vi "SaveReadoutToHDF5.vi"(7 "det_hardware":enum16{"CAMERA", "PMT"}(ring), 8 "error in":errorcluster, 9 "string seq in":string, 10 "readout":T1, 11 "File Paths":T2={"Local Save Path"=path "\\\\smbhome.uscs.susx.ac.uk\\cv222/Desktop/data", "Newton Save Path"=path "Z:/#Projects/Entanglement/data", "File Name"="test", "LocalSave"=TRUE}) -> (0 "error out":errorcluster, 3 "New data?":bool=TRUE)   [LabVIEW 2019]
uses:
  controls/FilePaths.ctl
  controls/GlobalExp.vi
  Global.lvlib
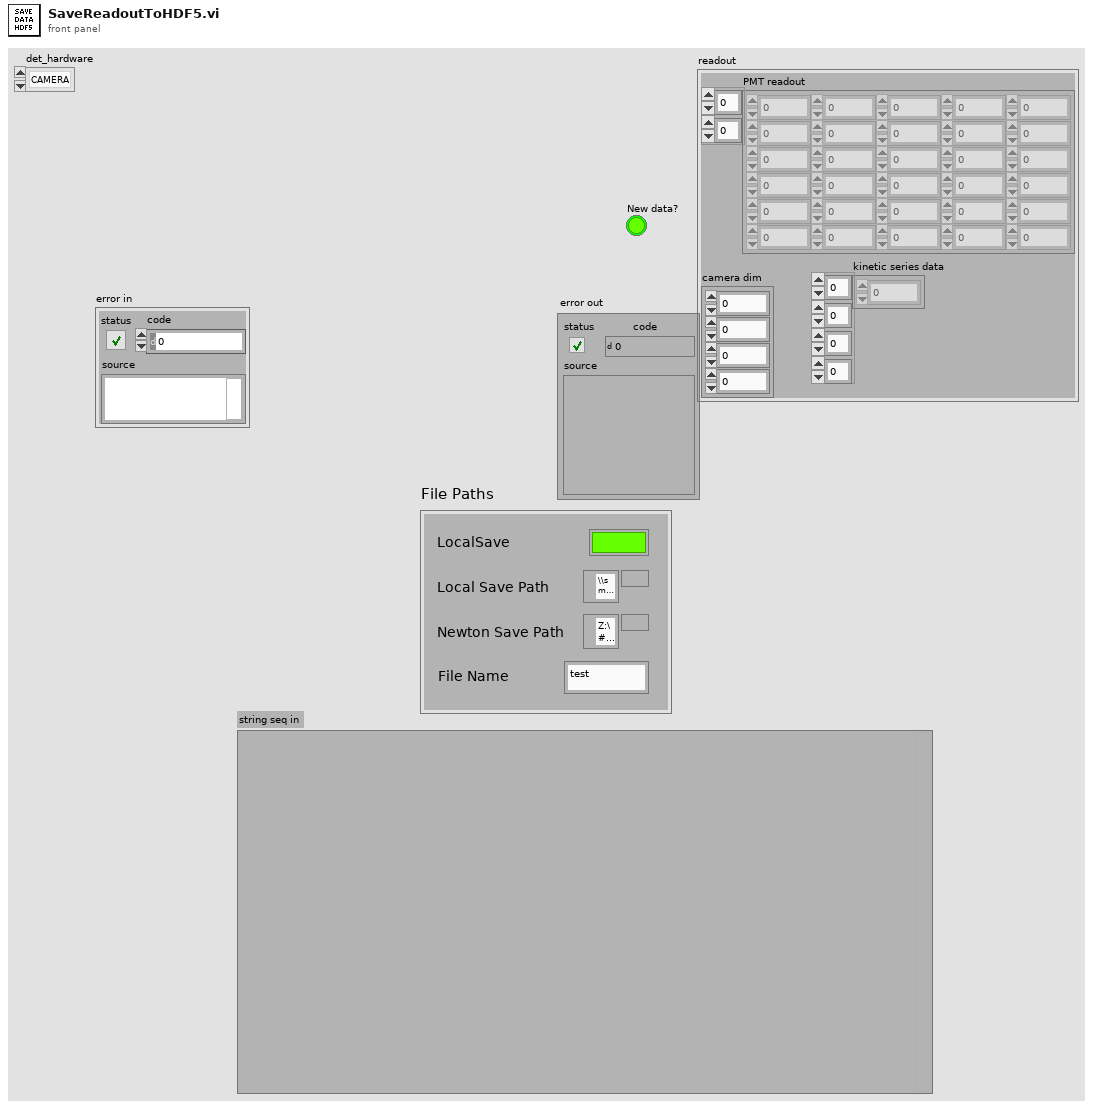
[diagram p1: front panel]
types:
  T1 = cluster{"PMT readout":u32[][], "kinetic series data":i32[][][][], "camera dim":cluster{i32, i32, i32, i32}}
  T2 = typedef "FilePaths.ctl" = cluster{"Local Save Path":path, "Newton Save Path":path, "File Name":string, "LocalSave":bool}
  T3 = cluster{"command":string, "steps":dbl, "runs":dbl, "det_hardware":string, "mathematica":string, "cam_dim":cluster{i32, i32, i32, i32}}
  T4 = typedef "MasterExpControl.ctl" = cluster{"Main Steps":dbl, "Main Runs":dbl, "ExpStatus":enum16{"Innit", "Stop", "Idle", "MainRunning", "AuxRunning"}, "Main Current Step":dbl, "ExpNum":dbl, "NewData":bool, "date":string, "command":string, "Stop":bool, "Pause":bool, "Mathematica":string, "Main/Meta":bool, "UpdateMath":bool, "Camera":bool, "MetaExpOver":bool, "NextMetaExp":bool}
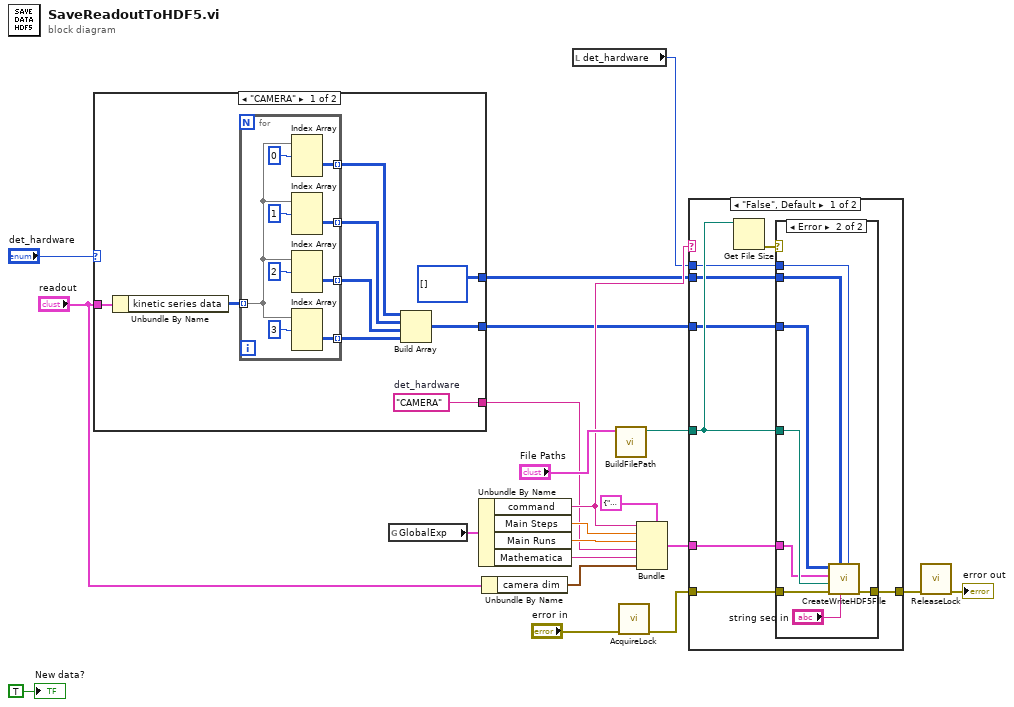
[diagram p0: block diagram]
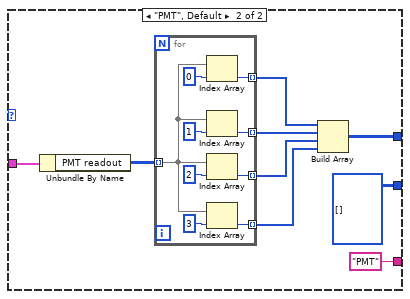
[diagram p2: hidden frame]
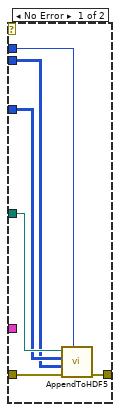
[diagram p3: hidden frame]
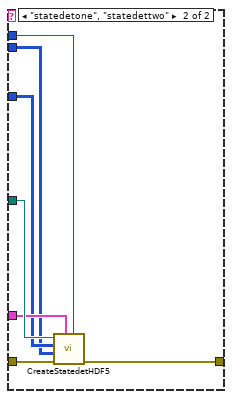
[diagram p4: hidden frame]
diagram:
  n1 = case shown="\"CAMERA\"" "det_hardware" {
    tunnel: "readout" -> [w25 w48]
    tunnel: [i16[][] [] w42] -> w6
    tunnel: [w26 i16[][][][] []] -> w5
    tunnel: [w22 "PMT" ("det_hardware")] -> w1
    frame "CAMERA" {
      w22 = "CAMERA"  # det_hardware
      n2 = Unbundle By Name(w25) -> ("kinetic series data"=w24:i32[][][][])
      n3 = for {
        tunnel: w24 -> [w35] mode=indexing
        tunnel: [w34] -> w30 mode=indexing
        tunnel: [w33] -> w29 mode=indexing
        tunnel: [w32] -> w28 mode=indexing
        tunnel: [w31] -> w27 mode=indexing
        n4 = Index Array(array=w35, index (dim 0)=0 ("index (page)")) -> (element=w34:i32[][])  [unwired: 2 in]
        n5 = Index Array(array=w35, index (dim 0)=1 ("index (page)")) -> (element=w33:i32[][])  [unwired: 2 in]
        n6 = Index Array(array=w35, index (dim 0)=2 ("index (page)")) -> (element=w32:i32[][])  [unwired: 2 in]
        n7 = Index Array(array=w35, index (dim 0)=3 ("index (page)")) -> (element=w31:i32[][])  [unwired: 2 in]
      }
      n8 = Build Array(w30, w29, w28, w27) -> (w26:i32[][][][])
    }
    frame "PMT", Default {
      n9 = Unbundle By Name(w48) -> ("PMT readout"=w47:u32[][])
      n10 = for {
        tunnel: w47 -> [w53] mode=indexing
        tunnel: [w52] -> w46 mode=indexing
        tunnel: [w51] -> w45 mode=indexing
        tunnel: [w50] -> w44 mode=indexing
        tunnel: [w49] -> w43 mode=indexing
        n11 = Index Array(array=w53, index=0 ("index (page)")) -> (element=w52:u32)
        n12 = Index Array(array=w53, index=1 ("index (page)")) -> (element=w51:u32)
        n13 = Index Array(array=w53, index=2 ("index (page)")) -> (element=w50:u32)
        n14 = Index Array(array=w53, index=3 ("index (page)")) -> (element=w49:u32)
      }
      n15 = Build Array(w46, w45, w44, w43) -> (w42:u32[][])
    }
  }
  n16 = global read "GlobalExp.vi" "GlobalExp"() -> (w21:T4)
  n17 = Unbundle By Name(w21) -> ("command"=w9:string, "Main Steps"=w12:dbl, "Main Runs"=w11:dbl, "Mathematica"=w10:string)
  n18 = Unbundle By Name("readout") -> ("camera dim"=w3:cluster{i32, i32, i32, i32})
  n19 = local read "det_hardware"() -> (w2:enum16{"CAMERA", "PMT"})
  n20 = call "BuildFilePath.vi"("File Paths"="File Paths") -> ("appended path"=w14:path)  [unwired: 10 in]
  n21 = call "AcquireLock.vi"("error in (no error)"="error in") -> ("error out"=w18:errorcluster)  [unwired: 10 in]
  n22 = Bundle(cluster=T3 {"command"="", "steps"=0.0, "runs"=0.0, "det_hardware"="", "mathematica"="", "cam_dim"={0, 0, 0, 0}}, "command"=w9, "steps"=w12, "runs"=w11, "det_hardware"=w1, "mathematica"=w10, "cam_dim"=w3) -> (w8:T3)
  n23 = case shown="\"False\", Default" w9 {
    tunnel: w14 -> [w64 w86]
    tunnel: w18 -> [w63 w85]
    tunnel: [w62 w84] -> w17
    tunnel: w6 -> [w61 w81]
    tunnel: w8 -> [w60 w83]
    tunnel: w5 -> [w59 w82]
    tunnel: w2 -> [w58 w80]
    frame "False", Default {
      n24 = Get File Size(file=w64) -> (0:w65:errorcluster)  [unwired: 1 in, 2 out]
      n25 = case shown="Error" w65 {
        tunnel: w64 -> [w71 w77]
        tunnel: w63 -> [w70 w78]
        tunnel: [w69 w79] -> w62
        tunnel: w60 -> [_ w76]
        tunnel: w61 -> [w66 w75]
        tunnel: w59 -> [w67 w74]
        tunnel: w58 -> [w68 w73]
        frame No Error {
          n26 = call "AppendToHDF5.vi"("det_hardware"=w68, "error in (no error)"=w70, "PMT IN"=w66, "Camera in"=w67, "appended path"=w71) -> ("error out"=w69:errorcluster)  [unwired: 6 in]
        }
        frame Error {
          n27 = call "CreateWriteHDF5File.vi"("Enum"=w73, "string seq in"="string seq in", "pmt data in"=w75, "error in (no error)"=w78, "path"=w77, "attributes"=w76, "Data in camera"=w74) -> ("error out"=w79:errorcluster)  [unwired: 4 in]
        }
      }
    }
    frame "statedetone", "statedettwo" {
      n28 = call "CreateStatedetHDF5.vi"("det_hardware"=w80, "attributes"=w83, "error in (no error)"=w85, "PMT readout"=w81, "kinetic series data"=w82, "appended path"=w86) -> ("error out"=w84:errorcluster)  [unwired: 5 in]
    }
  }
  n29 = call "ReleaseLock.vi"("error in (no error)"=w17) -> ("error out"=→"error out":errorcluster)  [unwired: 10 in]
  "New data?" <- TRUE ("Boolean")
